vi "Peter.vi"(9 "REPL":string, 10 "Send":string) -> ()   [LabVIEW 2020]
panel:
  out "Cover":bool
  in  "Script":string
  in  "Buffer":string
  in  "Disconnect":bool
  in  "EV3":T1={"EV3 IP Address"="192.168.1.93", "Username"="robot", "password"="maker"}
  in  "Help":bool
  in  "Connect":bool
  in  "Stop Button":bool
  out "Running Script":bool
  in  "Abort":bool
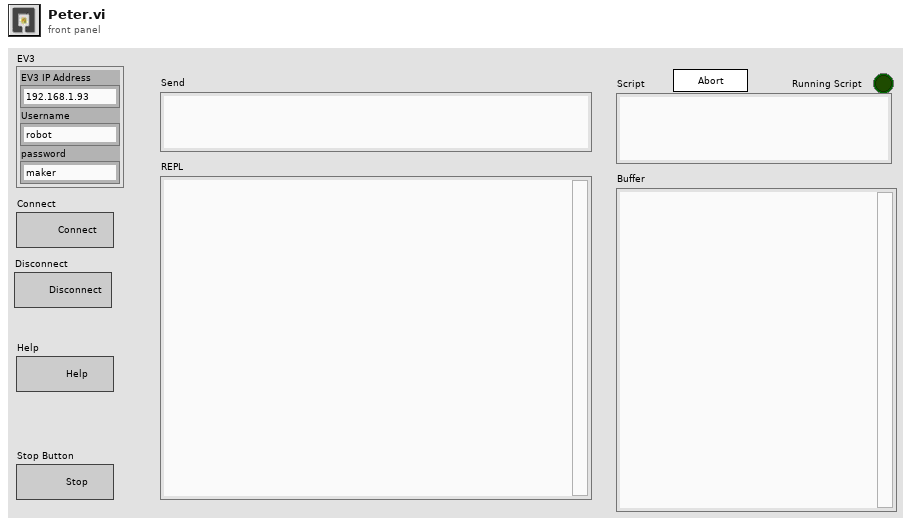
[diagram p1: front panel]
types:
  T1 = cluster{"EV3 IP Address":string, "Username":string, "password":string}
  T2 = enum32{"Invalid", "Standard", "Closed", "Hidden", "Minimized", "Maximized"}
  T3 = typedef "eventvkey.ctl" = enum16{"ASCII", "Enter", "Return", "Shift", "Ctrl", "Alt", "Cmd", "Opt", "Caps", "NumLock", "Clear", "Break", "Up", "Down", "Left", "Right", "Insert", "Delete", "Home", "End", "PageUp", "PageDown", "Escape", "Help", "Pause", "ScrollLock", "F1", "F2", "F3", "F4", "F5", "F6", "F7", "F8", "F9", "F10", "F11", "F12", "F13", "F14", "F15", "F16", "F17", "F18", "F19", "F20", "F21", "F22", "F23", "F24", "Play", "VolumeUp", "VolumeDown", "Mute", "Two Byte Char"}
  T4 = cluster{"Shift":bool, "Ctrl":bool, "Alt":bool, "Cmd":bool, "Opt":bool}
  T5 = cluster{"Char":i16, "VKey":T3, "PlatMods":cluster{"Shift":bool, "Ctrl":bool, "Alt":bool, "Cmd":bool, "Opt":bool}}
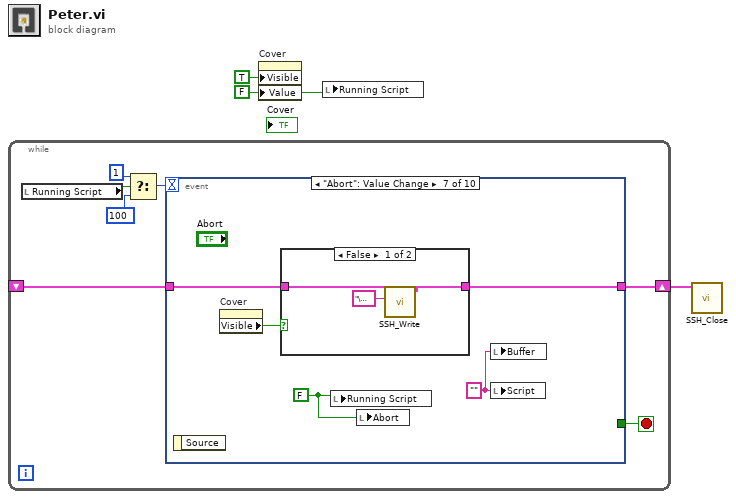
[diagram p0: block diagram]
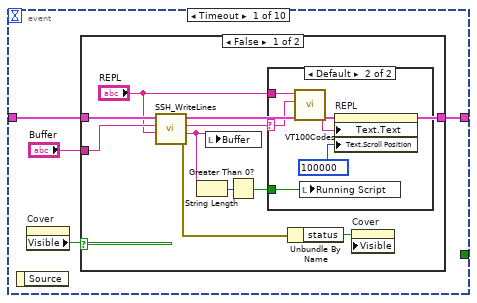
[diagram p2: hidden frame]
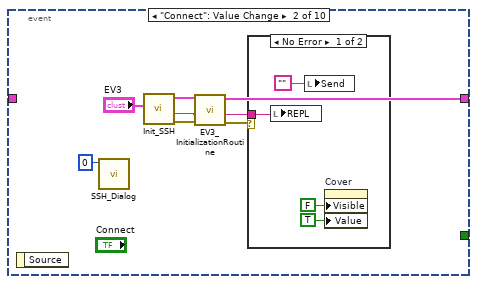
[diagram p5: hidden frame]
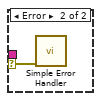
[diagram p6: hidden frame]
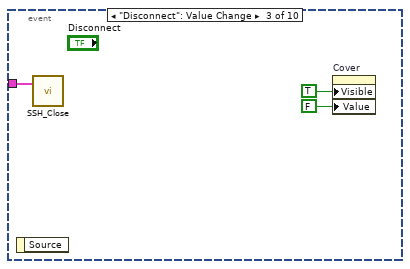
[diagram p7: hidden frame]
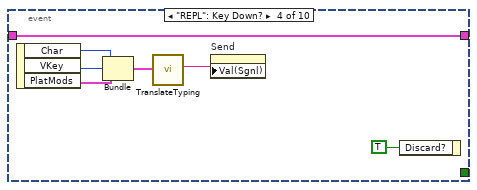
[diagram p8: hidden frame]
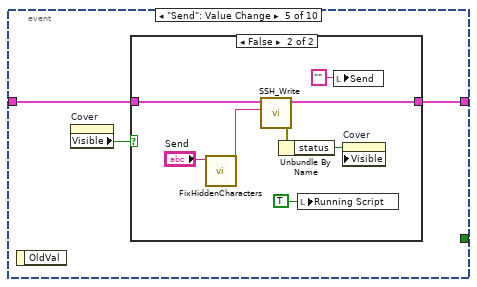
[diagram p9: hidden frame]
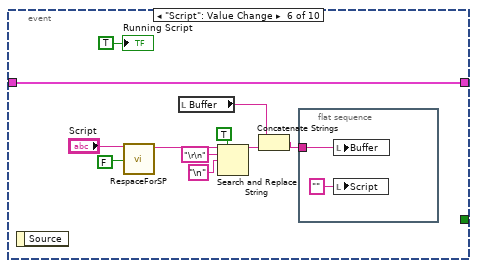
[diagram p11: hidden frame]
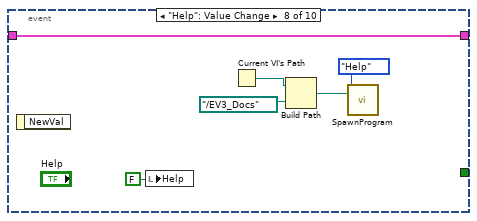
[diagram p13: hidden frame]
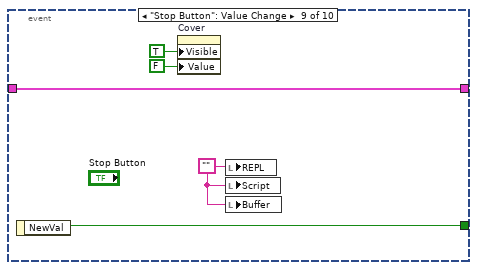
[diagram p14: hidden frame]
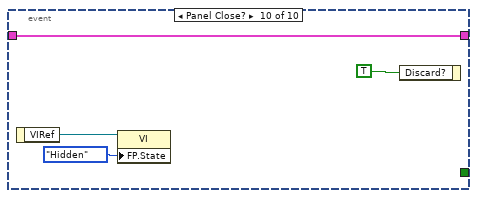
[diagram p15: hidden frame]
diagram:
  w1 = FALSE ("Cover")
  n1 = while {
    shift-right: [w9] -> w2
    shift-left: _ -> [w8]
    stop <- w10 stop-if-true
    n2 = local read "Running Script"() -> (w4:bool)
    n3 = Select(t=1, s=w4, f=100) -> (s? t:f=w5:i32)
    n4 = event shown="[6] \"Abort\": Value Change" {
      selector: _ -> [_ _ _ _ _ _ _ _ _ _]
      dyn-events: _ -> [_ _ _ _ _ _ _ _ _ _]
      timeout: w5 -> [_ _ _ _ _ _ _ _ _ _]
      tunnel: [_ _ _ _ _ _ _ _ w97 _] -> w10
      tunnel: [w14 w36 _ w52 w55 w76 w81 w93 w98 w102] -> w9
      tunnel: w8 -> [w12 _ w46 w52 w56 w76 w82 w93 w98 w102]
      event Timeout {
        n5 = event-data() -> ()  [unwired: 1 in, 1 out]
        n6 = property on="Cover" class="Bool (strict)"() -> ("Visible"=w13:bool)  [unwired: 2 in, 2 out]
        n7 = case shown="False" w13 {
          tunnel: [w21 w30] -> w14
          tunnel: w12 -> [w24 w30]
          tunnel: "Buffer" -> [w23 _]
          frame False {
            n8 = call "SSH_WriteLines.vi"("REPL"="REPL", "Buffer"=w23, "Python in"=w24) -> ("error out"=w18:errorcluster, "Rest"=w16:string, "Reply"=w20:string, "Python out"=w21:cluster{"Python":refnum<k35>, "py file":path})  [unwired: 5 in]
            n9 = String Length(string=w16) -> (length=w17:i32)
            n10 = local write "Buffer"(w16) -> ()
            n11 = Greater Than 0?(x=w17) -> (x > 0?=w15:bool)
            n12 = case shown="Default" w20 {
              selector: w20 -> [_ w26]
              tunnel: "REPL" -> [_ w27]
              tunnel: w15 -> [_ w25]
              frame "" {
              }
              frame Default {
                n13 = call "VT100Codes.vi"("read buffer"=w26, "Console In"=w27) -> ("Console Out"=w28:string)  [unwired: 9 in]
                n14 = local write "Running Script"(w25) -> ()
                n15 = property on="REPL" class="Str"("Text.Text"=w28, "Text.Scroll Position"=u32 100000 ("Text.Selection:Start")) -> ()  [unwired: 2 in, 2 out]
              }
            }
            n16 = Unbundle By Name(w18) -> ("status"=w22:bool)
            n17 = property on="Cover" class="Bool (strict)"("Visible"=w22) -> ()  [unwired: 2 in, 2 out]
          }
          frame True {
          }
        }
      }
      event "Connect": Value Change {
        n18 = event-data() -> ()  [unwired: 1 in, 1 out]
        n19 = call "SSH_Dialog.vi"("Slide"=u8 0) -> ()  [unwired: 11 in]
        n20 = call "Init_SSH.vi"("EV3"="EV3") -> ("error out"=w37:errorcluster, "Console out"=w32:string, "Python out"=w38:cluster{"Python":refnum<k35>, "py file":path})  [unwired: 8 in]
        n21 = call "EV3_InitializationRoutine.vi"("error in (no error)"=w37, "Console In"=w32, "Python in"=w38) -> ("error out"=w35:errorcluster, "Console Out"=w31:string, "Python out"=w36:cluster{"Python":refnum<k35>, "py file":path})  [unwired: 6 in]
        n22 = case shown="No Error" w35 {
          selector: w35 -> [_ w43]
          tunnel: w31 -> [w39 _]
          frame No Error {
            n23 = local write "REPL"(w39) -> ()
            n24 = local write "Send"("") -> ()
            n25 = property on="Cover" class="Bool (strict)"("Visible"=FALSE, "Value"=TRUE ("Cover")) -> ()  [unwired: 2 in, 2 out]
          }
          frame Error {
            n26 = call <vilib>:"Simple Error Handler.vi"("error in (no error)"=w43) -> ()  [unwired: 4 in, 5 out]
          }
        }
      }
      event "Disconnect": Value Change {
        n27 = event-data() -> ()  [unwired: 1 in, 1 out]
        n28 = call "SSH_Close.vi"("Python in"=w46) -> ()  [unwired: 11 in]
        n29 = property on="Cover" class="Bool (strict)"("Visible"=TRUE, "Value"=FALSE ("Cover")) -> ()  [unwired: 2 in, 2 out]
      }
      event "REPL": Key Down? {
        n30 = event-data() -> ("Char"=w50:i16, "VKey"=w49:T3, "PlatMods"=w48:T4)  [unwired: 1 in]
        n31 = Bundle("Char"=w50, "VKey"=w49, "PlatMods"=w48) -> (w51:T5)  [unwired: 1 in]
        n32 = call "TranslateTyping.vi"("Cluster"=w51) -> ("key"=w47:string)  [unwired: 10 in]
        n33 = property on="Send" class="Str"("Val(Sgnl)"=w47) -> ()  [unwired: 2 in, 2 out]
        n34 = event-data("Discard?"=TRUE) -> ()  [unwired: 1 in, 1 out]
      }
      event "Send": Value Change {
        n35 = event-data() -> ()  [unwired: 1 in, 1 out]
        n36 = property on="Cover" class="Bool (strict)"() -> ("Visible"=w54:bool)  [unwired: 2 in, 2 out]
        n37 = case shown="False" w54 {
          tunnel: w56 -> [w57 w63]
          tunnel: [w57 w62] -> w55
          frame True {
          }
          frame False {
            n38 = call "FixHiddenCharacters.vi"("String in"="Send") -> ("String out"=w59:string)  [unwired: 10 in]
            n39 = call "SSH_Write.vi"("Text to write"=w59, "Python in"=w63) -> ("error out"=w61:errorcluster, "Python out"=w62:cluster{"Python":refnum<k35>, "py file":path})  [unwired: 8 in]
            n40 = Unbundle By Name(w61) -> ("status"=w64:bool)
            n41 = local write "Running Script"(TRUE ("Running Script")) -> ()
            n42 = local write "Send"("" ("Write text")) -> ()
            n43 = property on="Cover" class="Bool (strict)"("Visible"=w64) -> ()  [unwired: 2 in, 2 out]
          }
        }
      }
      event "Script": Value Change {
        n44 = event-data() -> ()  [unwired: 1 in, 1 out]
        n45 = call "RespaceForSP.vi"("Keep spaces?"=FALSE, "Code"="Script") -> ("Cleaned for SPIKE"=w71:string)  [unwired: 9 in]
        n46 = local read "Buffer"() -> (w68:string)
        n47 = Search and Replace String(replace all?=TRUE ("replace all? (F)"), input string=w71, search string="\r\n", replace string="\n" ("search string")) -> (result string=w67:string)  [unwired: 4 in, 3 out]
        n48 = Concatenate Strings(w68, w67) -> (w66:string)
        n49 = flat-sequence {
          tunnel: w66 -> [w78]
          frame #0 {
            n50 = local write "Buffer"(w78) -> ()
            n51 = local write "Script"("" ("Script")) -> ()
          }
        }
        "Running Script" <- TRUE ("Running Script")
      }
      event "Abort": Value Change {
        w83 = "" ("Script")
        w80 = FALSE ("Running Script")
        n52 = event-data() -> ()  [unwired: 1 in, 1 out]
        n53 = property on="Cover" class="Bool (strict)"() -> ("Visible"=w79:bool)  [unwired: 2 in, 2 out]
        n54 = case shown="False" w79 {
          tunnel: w82 -> [w86 w87]
          tunnel: [w85 w87] -> w81
          frame False {
            n55 = call "SSH_Write.vi"("Text to write"="\u0003", "Python in"=w86) -> ("Python out"=w85:cluster{"Python":refnum<k35>, "py file":path})  [unwired: 8 in, 1 out]
          }
          frame True {
          }
        }
        n56 = local write "Running Script"(w80) -> ()
        n57 = local write "Abort"(w80) -> ()
        n58 = local write "Buffer"(w83) -> ()
        n59 = local write "Script"(w83) -> ()
      }
      event "Help": Value Change {
        n60 = event-data() -> ()  [unwired: 1 in, 1 out]
        n61 = local write "Help"(FALSE ("Help")) -> ()
        n62 = Current VI's Path() -> (path=w91:path)
        n63 = Build Path(base path=w91, name or relative path=path "../EV3_Docs") -> (appended path=w88:path)
        n64 = call "SpawnProgram.vi"("Server"=w88, "Dialog"=enum16{"Help", "Files"}."Help") -> ()  [unwired: 10 in]
      }
      event "Stop Button": Value Change {
        w94 = ""
        n65 = event-data() -> ("NewVal"=w97:bool)  [unwired: 1 in]
        n66 = property on="Cover" class="Bool (strict)"("Visible"=TRUE, "Value"=FALSE ("Cover")) -> ()  [unwired: 2 in, 2 out]
        n67 = local write "REPL"(w94) -> ()
        n68 = local write "Script"(w94) -> ()
        n69 = local write "Buffer"(w94) -> ()
      }
      event Panel Close? {
        n70 = event-data() -> ("VIRef"=w100:refnum<vi>)  [unwired: 1 in]
        n71 = property class="VI"(reference=w100, "FP.State"=T2."Hidden" ("Front Panel Window:State")) -> ()  [unwired: 1 in, 2 out]
        n72 = event-data("Discard?"=TRUE) -> ()  [unwired: 1 in, 1 out]
      }
    }
  }
  n73 = property on="Cover" class="Bool (strict)"("Visible"=TRUE, "Value"=w1) -> ()  [unwired: 2 in, 2 out]
  n74 = local write "Running Script"(w1) -> ()
  n75 = call "SSH_Close.vi"("Python in"=w2) -> ()  [unwired: 11 in]
